vi "Load config.vi"(8 "error in (no error)":errorcluster) -> (0 "error out":errorcluster, 3 "DAQ Port":tag)   [LabVIEW 2020]
uses:
  <vilib>/Utility/config.llb/NI_LVConfig.lvlib
  <vilib>/Utility/config.llb/Read Key (String).vi
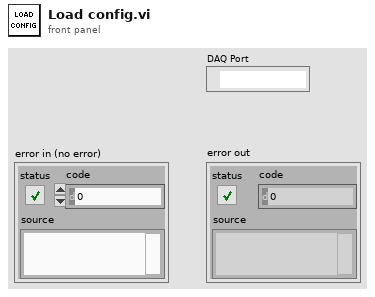
[diagram p1: front panel]
types:
  T1 = typedef "NI_LVConfig.lvlib/Config Data RefNum.ctl" = refnum<k1>
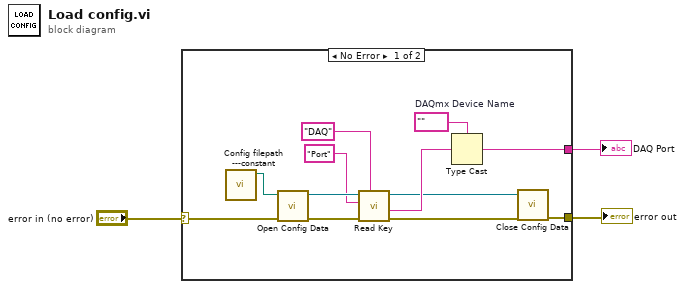
[diagram p0: block diagram]
diagram:
  n1 = case shown="No Error" "error in (no error)" {
    selector: "error in (no error)" -> [w14 w16]
    tunnel: [w7 w16] -> w2
    tunnel: [w5 _] -> w1
    frame No Error {
      w6 = tag ""  # DAQmx Device Name
      n2 = call "Config filepath ---constant.vi"() -> ("config file path"=w15:path)  [unwired: 11 in]
      n3 = call <vilib>:"Open Config Data.vi"("error in (no error)"=w14, "configuration file path"=w15) -> ("error out"=w12:errorcluster, "refnum"=w13:T1)  [unwired: 7 in, 1 out]
      n4 = call-poly <vilib>:"Read Key.vi"("section"="DAQ", "error in (no error)"=w12, "key"="Port", "refnum"=w13) -> ("error out"=w8:errorcluster, "value"=w10:string, "refnum out"=w9:T1)  [unwired: 4 in, 1 out]
      n5 = Type Cast(type=w6, x=w10) -> (*(type *) &x=w5:tag)
      n6 = call <vilib>:"Close Config Data.vi"("error in (no error)"=w8, "refnum"=w9) -> ("error out"=w7:errorcluster)  [unwired: 8 in, 1 out]
    }
    frame Error {
    }
  }
  "error out" <- w2
  "DAQ Port" <- w1
